vi "Data_Save_BOOST.vi"(9 "Data":T1) -> (2 "BOOST":string[](array[string]))   [LabVIEW 2017]
uses:
  Ctrls/Data.ctl
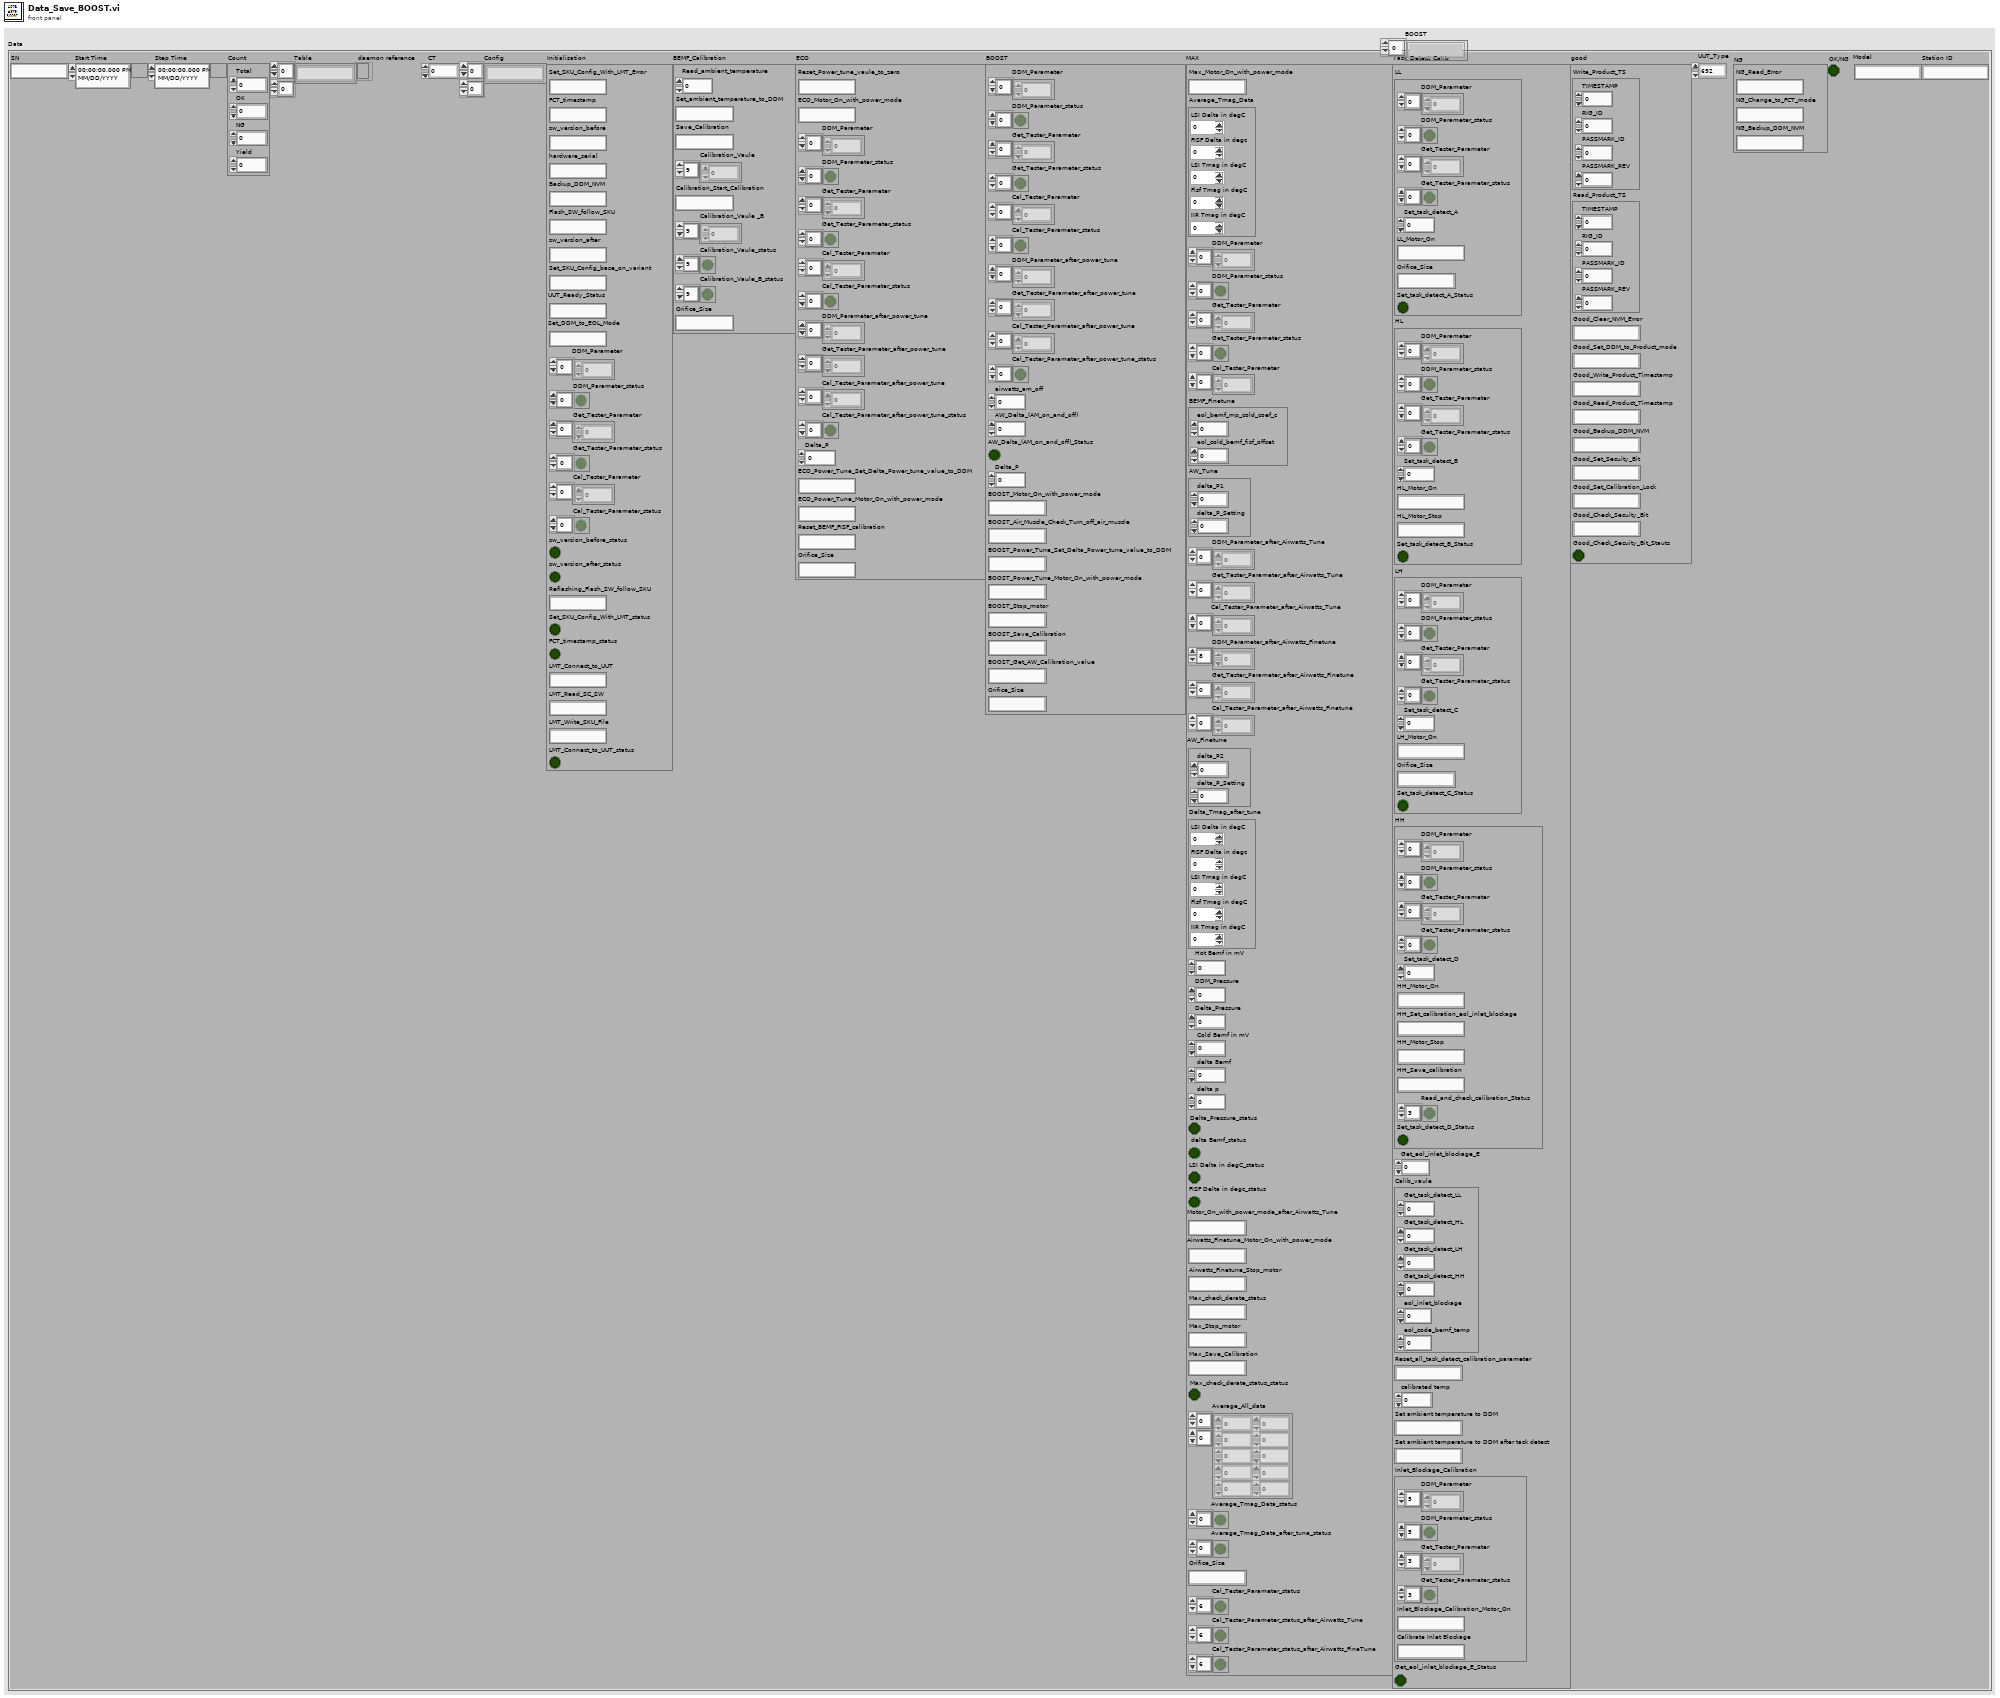
[diagram p1: front panel]
types:
  T1 = typedef "Data.ctl" = cluster{"SN":string, "Start Time":timestamp, "Step Time":timestamp, "Count":cluster{"Total":i32, "OK":i32, "NG":i32, "Yield":dbl}, "Table":string[][], "daemon reference":refnum<k5>, "CT":dbl, "Config":string[][], "Initialisation":cluster{"Set_SKU_Config_With_LMT_Error":string, "FCT_timestamp":string, "sw_version_before":string, "hardware_serial":string, "Backup_DDM_NVM":string, "Flash_SW_follow_SKU":string, "sw_version_after":string, "Set_SKU_Config_base_on_variant":string, "UUT_Ready_Status":string, "Set_DDM_to_EOL_Mode":string, "DDM_Parameter":dbl[], "DDM_Parameter_status":bool[], "Get_Tester_Parameter":dbl[], "Get_Tester_Parameter_status":bool[], "Cal_Tester_Parameter":dbl[], "Cal_Tester_Parameter_status":bool[], "sw_version_before_status":bool, "sw_version_after_status":bool, "Reflashing_Flash_SW_follow_SKU":string, "Set_SKU_Config_With_LMT_status":bool, "FCT_timestamp_status":bool, "LMT_Connect_to_UUT":string, "LMT_Read_SC_SW":string, "LMT_Write_SKU_File":string, "LMT_Connect_to_UUT_status":bool}, "BEMF_Calibration":cluster{"Read_ambient_temperature":dbl, "Set_ambient_temperature_to_DDM":string, "Save_Calibration":string, "Calibration_Vaule":dbl[], "Calibration_Start_Calibration":string, "Calibration_Vaule _B":dbl[], "Calibration_Vaule_status":bool[], "Calibration_Vaule_B_status":bool[], "Orifice_Size":string}, "ECO":cluster{"Reset_Power_tune_vaule_to_zero":string, "ECO_Motor_On_with_power_mode":string, "DDM_Parameter":dbl[], "DDM_Parameter_status":bool[], "Get_Tester_Parameter":dbl[], "Get_Tester_Parameter_status":bool[], "Cal_Tester_Parameter":dbl[], "Cal_Tester_Parameter_status":bool[], "DDM_Parameter_after_power_tune":dbl[], "Get_Tester_Parameter_after_power_tune":dbl[], "Cal_Tester_Parameter_after_power_tune":dbl[], "Cal_Tester_Parameter_after_power_tune_status":bool[], "Delta_P":dbl, "ECO_Power_Tune_Set_Delta_Power_tune_value_to_DDM":string, "ECO_Power_Tune_Motor_On_with_power_mode":string, "Reset_BEMF_FISF_calibration":string, "Orifice_Size":string}, "BOOST":cluster{"DDM_Parameter":dbl[], "DDM_Parameter_status":bool[], "Get_Tester_Parameter":dbl[], "Get_Tester_Parameter_status":bool[], "Cal_Tester_Parameter":dbl[], "Cal_Tester_Parameter_status":bool[], "DDM_Parameter_after_power_tune":dbl[], "Get_Tester_Parameter_after_power_tune":dbl[], "Cal_Tester_Parameter_after_power_tune":dbl[], "Cal_Tester_Parameter_after_power_tune_status":bool[], "airwatts_am_off":dbl, "AW_Delta_(AM_on_and_off)":dbl, "AW_Delta_(AM_on_and_off)_Status":bool, "Delta_P":dbl, "BOOST_Motor_On_with_power_mode":string, "BOOST_Air_Muscle_Check_Turn_off_air_muscle":string, "BOOST_Power_Tune_Set_Delta_Power_tune_value_to_DDM":string, "BOOST_Power_Tune_Motor_On_with_power_mode":string, "BOOST_Stop_motor":string, "BOOST_Save_Calibration":string, "BOOST_Get_AW_Calibration_value":string, "Orifice_Size":string}, "MAX":cluster{"Max_Motor_On_with_power_mode":string, "Average_Tmag_Data":cluster{"LSI Delta in degC":dbl, "FISF Delta in degc":dbl, "LSI Tmag in degC":dbl, "Fisf Tmag in degC":dbl, "IIR Tmag in degC":dbl}, "DDM_Parameter":dbl[], "DDM_Parameter_status":bool[], "Get_Tester_Parameter":dbl[], "Get_Tester_Parameter_status":bool[], "Cal_Tester_Parameter":dbl[], "BEMF_Finetune":cluster{"eol_bemf_mp_cold_coef_c":dbl, "eol_cold_bemf_fisf_offset":dbl}, "AW_Tune":cluster{"delta_P1":dbl, "delta_P_Setting":dbl}, "DDM_Parameter_after_Airwatts_Tune":dbl[], "Get_Tester_Parameter_after_Airwatts_Tune":dbl[], "Cal_Tester_Parameter_after_Airwatts_Tune":dbl[], "DDM_Parameter_after_Airwatts_Finetune":dbl[], "Get_Tester_Parameter_after_Airwatts_Finetune":dbl[], "Cal_Tester_Parameter_after_Airwatts_Finetune":dbl[], "AW_Finetune":cluster{"delta_P2":dbl, "delta_P_Setting":dbl}, "Delta_Tmag_after_tune":cluster{"LSI Delta in degC":dbl, "FISF Delta in degc":dbl, "LSI Tmag in degC":dbl, "Fisf Tmag in degC":dbl, "IIR Tmag in degC":dbl}, "Hot Bemf in mV":dbl, "DDM_Pressure":dbl, "Delta_Pressure":dbl, " Cold Bemf in mV":dbl, " delta Bemf":dbl, " delta p":dbl, "Delta_Pressure_status":bool, " delta Bemf_status":bool, "LSI Delta in degC_status":bool, "FISF Delta in degc_status":bool, "Motor_On_with_power_mode_after_Airwatts_Tune":string, "Airwatts_Finetune_Motor_On_with_power_mode":string, "Airwatts_Finetune_Stop_motor":string, "Max_check_derate_status":string, "Max_Stop_motor":string, "Max_Save_Calibration":string, "Max_check_derate_status_status":bool, "Average_All_data":dbl[][], "Average_Tmag_Data_status":bool[], "Average_Tmag_Data_after_tune_status":bool[], "Orifice_Size":string, "Cal_Tester_Parameter_status":bool[], "Cal_Tester_Parameter_status_after_Airwatts_Tune":bool[], "Cal_Tester_Parameter_status_after_Airwatts_FineTune":bool[]}, "Task_Detect_Calib":cluster{"LL":cluster{"DDM_Parameter":dbl[], "DDM_Parameter_status":bool[], "Get_Tester_Parameter":dbl[], "Get_Tester_Parameter_status":bool[], "Set_task_detect_A":dbl, "LL_Motor_On":string, "Orifice_Size":string, "Set_task_detect_A_Status":bool}, "HL":cluster{"DDM_Parameter":dbl[], "DDM_Parameter_status":bool[], "Get_Tester_Parameter":dbl[], "Get_Tester_Parameter_status":bool[], "Set_task_detect_B":dbl, "HL_Motor_On":string, "HL_Motor_Stop":string, "Set_task_detect_B_Status":bool}, "LH":cluster{"DDM_Parameter":dbl[], "DDM_Parameter_status":bool[], "Get_Tester_Parameter":dbl[], "Get_Tester_Parameter_status":bool[], "Set_task_detect_C":dbl, "LH_Motor_On":string, "Orifice_Size":string, "Set_task_detect_C_Status":bool}, "HH":cluster{"DDM_Parameter":dbl[], "DDM_Parameter_status":bool[], "Get_Tester_Parameter":dbl[], "Get_Tester_Parameter_status":bool[], "Set_task_detect_D":dbl, "HH_Motor_On":string, "HH_Set_calibration_eol_inlet_blockage":string, "HH_Motor_Stop":string, "HH_Save_calibration":string, "Read_and_check_calibration_Status":bool[], "Set_task_detect_D_Status":bool}, "Get_eol_inlet_blockage_E":dbl, "Calib_vaule":cluster{"Get_task_detect_LL":dbl, "Get_task_detect_HL":dbl, "Get_task_detect_LH":dbl, "Get_task_detect_HH":dbl, "eol_inlet_blockage":dbl, "eol_code_bemf_temp":dbl}, "Reset_all_task_detect_calibration_parameter":string, "calibrated temp":dbl, "Set ambient temperature to DDM":string, "Set ambient temperature to DDM after task detect":string, "Inlet_Blockage_Calibration":cluster{"DDM_Parameter":dbl[], "DDM_Parameter_status":bool[], "Get_Tester_Parameter":dbl[], "Get_Tester_Parameter_status":bool[], "Inlet_Blockage_Calibration_Motor_On":string, "Calibrate Inlet Blockage":string}, "Get_eol_inlet_blockage_E_Status":bool}, "good":cluster{"Write_Product_TS":cluster{"TIMESTAMP":i64, "RIG_ID":i64, "PASSMARK_ID":i64, "PASSMARK_REV":i64}, "Read_Product_TS":cluster{"TIMESTAMP":i64, "RIG_ID":i64, "PASSMARK_ID":i64, "PASSMARK_REV":i64}, "Good_Clear_NVM_Error":string, "Good_Set_DDM_to_Product_mode":string, "Good_Write_Product_Timestamp":string, "Good_Read_Product_Timestamp":string, "Good_Backup_DDM_NVM":string, "Good_Set_Secuity_Bit":string, "Good_Set_Calibration_Lock":string, "Good_Check_Secuity_Bit":string, "Good_Check_Secuity_Bit_Stauts":bool}, "UUT_Type":enum16{"692", "692B", "692D"}, "NG":cluster{"NG_Read_Error":string, "NG_Change_to_FCT_mode":string, "NG_Backup_DDM_NVM":string}, "OK/NG":bool, "Model":string, "Station ID":string}
  T2 = typedef "HD Config.ctl" = cluster{" PC":cluster{"PC Address":u8[], "PC Port":i32}, "FCO":cluster{"COM":refnum<visa-resource-name>, "Baudrate":u32}, "DC Power ":cluster{"COM":refnum<visa-resource-name>, "Baudrate":u32}, "PW3336":cluster{"COM":refnum<visa-resource-name>, "Baudrate":u32}, "Lefoo":cluster{"COM":refnum<visa-resource-name>, "Baudrate":u32}, "AI Model":cluster{"COM":refnum<visa-resource-name>, "Baudrate":u32}, "DIPC":cluster{"COM":refnum<visa-resource-name>}, "Daemon":cluster{"IP Address":string, "Port":u16, "Retry":u16}, "Motor":cluster{"COM":refnum<visa-resource-name>, "Baudrate":u32}, "G1":bool, "Fail_resume_mode":bool, "Skip DDM Speed&Pressure Passmark":bool}
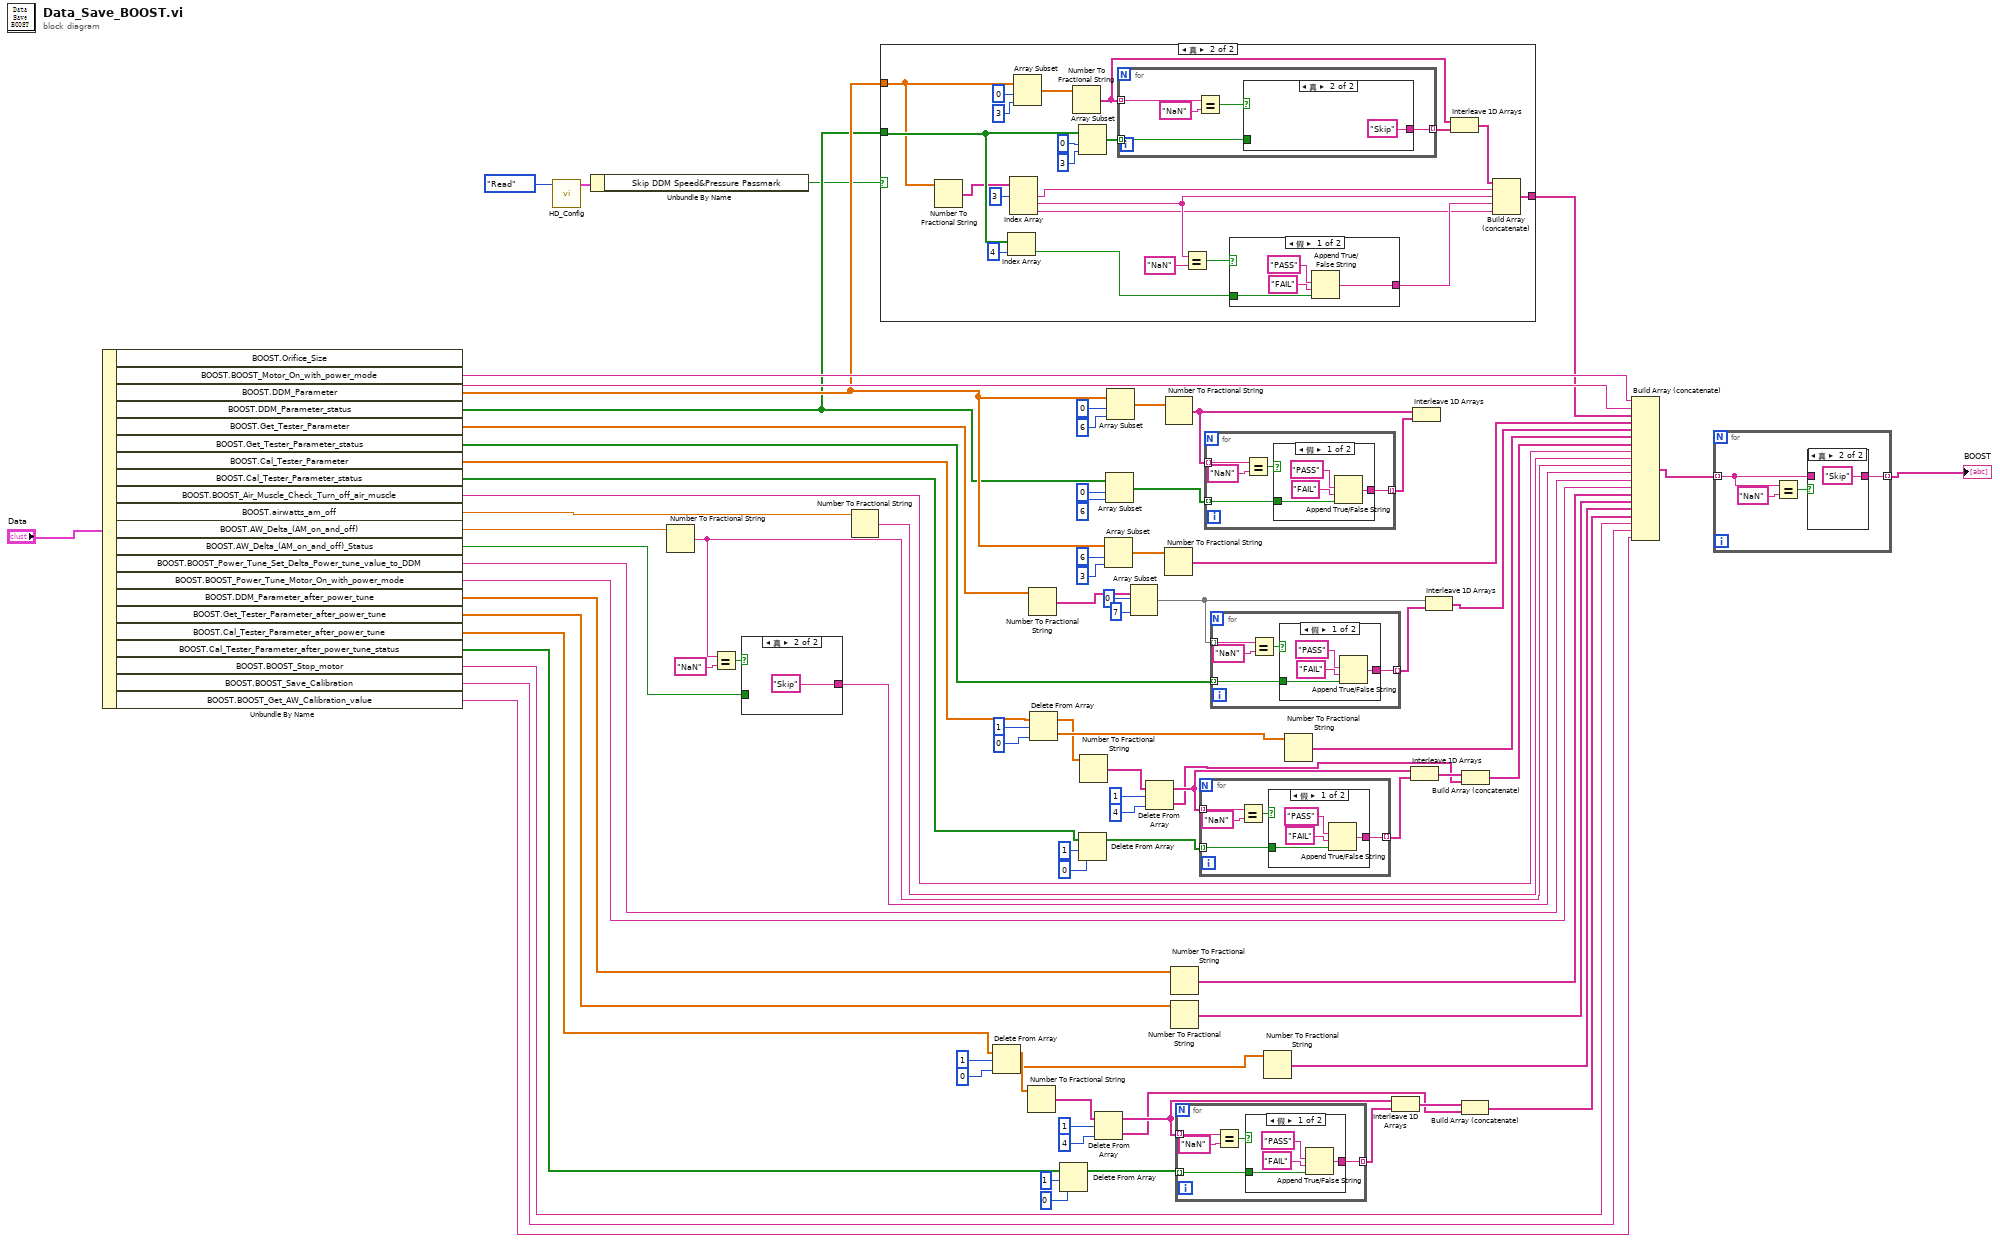
[diagram p0: block diagram]
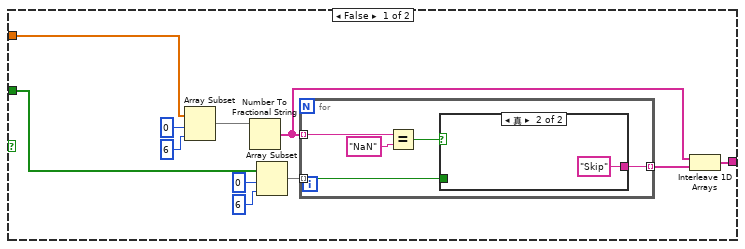
[diagram p2: hidden frame]
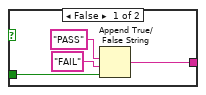
[diagram p3: hidden frame]
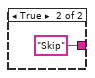
[diagram p4: hidden frame]
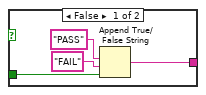
[diagram p5: hidden frame]
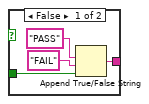
[diagram p6: hidden frame]
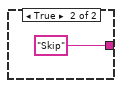
[diagram p8: hidden frame]
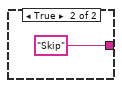
[diagram p9: hidden frame]
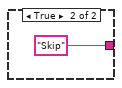
[diagram p10: hidden frame]
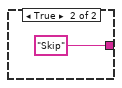
[diagram p11: hidden frame]
diagram:
  n1 = Unbundle By Name("Data") -> ("BOOST.Orifice_Size"=w25:string, "BOOST.BOOST_Motor_On_with_power_mode"=w26:string, "BOOST.DDM_Parameter"=w24:dbl[], "BOOST.DDM_Parameter_status"=w23:bool[], "BOOST.Get_Tester_Parameter"=w14:dbl[], "BOOST.Get_Tester_Parameter_status"=w38:bool[], "BOOST.Cal_Tester_Parameter"=w65:dbl[], "BOOST.Cal_Tester_Parameter_status"=w64:bool[], "BOOST.BOOST_Air_Muscle_Check_Turn_off_air_muscle"=w51:string, "BOOST.airwatts_am_off"=w50:dbl, "BOOST.AW_Delta_(AM_on_and_off)"=w49:dbl, "BOOST.AW_Delta_(AM_on_and_off)_Status"=w29:bool, "BOOST.BOOST_Power_Tune_Set_Delta_Power_tune_value_to_DDM"=w47:string, "BOOST.BOOST_Power_Tune_Motor_On_with_power_mode"=w46:string, "BOOST.DDM_Parameter_after_power_tune"=w81:dbl[], "BOOST.Get_Tester_Parameter_after_power_tune"=w82:dbl[], "BOOST.Cal_Tester_Parameter_after_power_tune"=w55:dbl[], "BOOST.Cal_Tester_Parameter_after_power_tune_status"=w54:bool[], "BOOST.BOOST_Stop_motor"=w45:string, "BOOST.BOOST_Save_Calibration"=w44:string, "BOOST.BOOST_Get_AW_Calibration_value"=w43:string)
  n2 = call "HD_Config.vi"("Step"=enum16{"Initial", "Write", "Read"}."Read") -> ("HD Config out"=w20:T2)  [unwired: 9 in, 1 out]
  n3 = Unbundle By Name(w20) -> ("Skip DDM Speed&Pressure Passmark"=w19:bool)
  n4 = Number To Fractional String(number=w49) -> (F-format string=w28:string)  [unwired: 3 in]
  n5 = Equal?(x=w28, y="NaN" ("x")) -> (x = y?=w30:bool)
  n6 = case shown="真" w30 {
    tunnel: w29 -> [w89 _]
    tunnel: [w87 "Skip" ("x")] -> w27
    frame False {
      n7 = Append True/False String(1:w89, 2:"FAIL" ("字符串(\"\")"), 3:"PASS" ("真字符串")) -> (0:w87:string)  [unwired: 1 in]
    }
    frame True {
    }
  }
  n8 = Number To Fractional String(number=w50) -> (F-format string=w48:string)  [unwired: 3 in]
  n9 = case shown="真" w19 {
    tunnel: w23 -> [w92 w123]
    tunnel: w24 -> [w93 w120]
    tunnel: [w91 w112] -> w22
    frame False {
      n10 = Array Subset(array=w93, index=0 ("索引"), length=6 ("长度")) -> (w99:dbl[])
      n11 = Number To Fractional String(number=w99) -> (F-format string=w98:string[])  [unwired: 3 in]
      n12 = Array Subset(array=w92, index=0 ("索引"), length=6 ("长度")) -> (w100:bool[])
      n13 = for {
        tunnel: w100 -> [w106] mode=indexing
        tunnel: [w105] -> w101 mode=indexing
        tunnel: w98 -> [w103] mode=indexing
        n14 = Equal?(x=w103, y="NaN" ("x")) -> (x = y?=w102:bool)
        n15 = case shown="真" w102 {
          tunnel: w106 -> [w110 _]
          tunnel: [w108 "Skip" ("x")] -> w105
          frame False {
            n16 = Append True/False String(1:w110, 2:"FAIL" ("字符串(\"\")"), 3:"PASS" ("真字符串")) -> (0:w108:string)  [unwired: 1 in]
          }
          frame True {
          }
        }
      }
      n17 = Interleave 1D Arrays(w98, w101) -> (w91:string[])
    }
    frame True {
      n18 = Number To Fractional String(number=w120) -> (F-format string=w119:string[])  [unwired: 3 in]
      n19 = Index Array(array=w123, index=4 ("索引")) -> (element=w118:bool)
      n20 = Index Array(array=w119, index #1=3 ("索引")) -> (element #1=w117:string, element #2=w115:string, element #3=w114:string)  [unwired: 2 in]
      n21 = Array Subset(array=w120, index=0 ("索引"), length=3 ("长度")) -> (w131:dbl[])
      n22 = Number To Fractional String(number=w131) -> (F-format string=w126:string[])  [unwired: 3 in]
      n23 = Array Subset(array=w123, index=0 ("索引"), length=3 ("长度")) -> (w132:bool[])
      n24 = for {
        tunnel: w132 -> [w143] mode=indexing
        tunnel: [w142] -> w133 mode=indexing
        tunnel: w126 -> [w140] mode=indexing
        n25 = Equal?(x=w140, y="NaN" ("x")) -> (x = y?=w139:bool)
        n26 = case shown="真" w139 {
          tunnel: w143 -> [w147 _]
          tunnel: [w145 "Skip" ("x")] -> w142
          frame False {
            n27 = Append True/False String(1:w147, 2:"FAIL" ("字符串(\"\")"), 3:"PASS" ("真字符串")) -> (0:w145:string)  [unwired: 1 in]
          }
          frame True {
          }
        }
      }
      n28 = Equal?(x=w115, y="NaN" ("x")) -> (x = y?=w122:bool)
      n29 = case shown="假" w122 {
        tunnel: w118 -> [w137 _]
        tunnel: [w135 "Skip" ("x")] -> w116
        frame False {
          n30 = Append True/False String(1:w137, 2:"FAIL" ("字符串(\"\")"), 3:"PASS" ("真字符串")) -> (0:w135:string)  [unwired: 1 in]
        }
        frame True {
        }
      }
      n31 = Interleave 1D Arrays(w126, w133) -> (w113:string[])
      n32 = Build Array (concatenate)(w113, w117, w115, w116, w114) -> (w112:string[])
    }
  }
  n33 = Delete From Array(array=w55, length=1 ("长度"), index=0 ("索引")) -> (deleted portion=w58:dbl[], array with subset deleted=w59:dbl[])
  n34 = Number To Fractional String(number=w59) -> (F-format string=w4:string[])  [unwired: 3 in]
  n35 = Number To Fractional String(number=w14) -> (F-format string=w15:string[])  [unwired: 3 in]
  n36 = Delete From Array(array=w65, length=1 ("长度"), index=0 ("索引")) -> (deleted portion=w69:dbl[], array with subset deleted=w68:dbl[])
  n37 = Delete From Array(array=w54, length=1 ("长度"), index=0 ("索引")) -> (array with subset deleted=w35:bool[])  [unwired: 1 out]
  n38 = Delete From Array(array=w64, length=1 ("长度"), index=0 ("索引")) -> (array with subset deleted=w36:bool[])  [unwired: 1 out]
  n39 = Number To Fractional String(number=w68) -> (F-format string=w11:string[])  [unwired: 3 in]
  n40 = Delete From Array(array=w4, length=1 ("长度"), index=4 ("索引")) -> (deleted portion=w1:string[], array with subset deleted=w3:string[])
  n41 = Array Subset(array=w24, index=6 ("索引"), length=3 ("长度")) -> (w73:dbl[])
  n42 = Array Subset(array=w23, index=0 ("索引"), length=6 ("长度")) -> (w41:bool[])
  n43 = Array Subset(array=w24, index=0 ("索引"), length=6 ("长度")) -> (w74:dbl[])
  n44 = Array Subset(array=w15, index=0 ("索引"), length=7 ("长度")) -> (w18:string[])
  n45 = Delete From Array(array=w11, length=1 ("长度"), index=4 ("索引")) -> (deleted portion=w8:string[], array with subset deleted=w10:string[])
  n46 = Number To Fractional String(number=w73) -> (F-format string=w83:string[])  [unwired: 3 in]
  n47 = Number To Fractional String(number=w74) -> (F-format string=w40:string[])  [unwired: 3 in]
  n48 = Number To Fractional String(number=w81) -> (F-format string=w84:string[])  [unwired: 3 in]
  n49 = Number To Fractional String(number=w82) -> (F-format string=w85:string[])  [unwired: 3 in]
  n50 = for {
    tunnel: w35 -> [w153] mode=indexing
    tunnel: [w152] -> w34 mode=indexing
    tunnel: w3 -> [w150] mode=indexing
    n51 = Equal?(x=w150, y="NaN" ("x")) -> (x = y?=w149:bool)
    n52 = case shown="假" w149 {
      tunnel: w153 -> [w157 _]
      tunnel: [w155 "Skip" ("x")] -> w152
      frame False {
        n53 = Append True/False String(1:w157, 2:"FAIL" ("字符串(\"\")"), 3:"PASS" ("真字符串")) -> (0:w155:string)  [unwired: 1 in]
      }
      frame True {
      }
    }
  }
  n54 = for {
    tunnel: w36 -> [w163] mode=indexing
    tunnel: [w162] -> w37 mode=indexing
    tunnel: w10 -> [w160] mode=indexing
    n55 = Equal?(x=w160, y="NaN" ("x")) -> (x = y?=w159:bool)
    n56 = case shown="假" w159 {
      tunnel: w163 -> [w167 _]
      tunnel: [w165 "Skip" ("x")] -> w162
      frame False {
        n57 = Append True/False String(1:w167, 2:"FAIL" ("字符串(\"\")"), 3:"PASS" ("真字符串")) -> (0:w165:string)  [unwired: 1 in]
      }
      frame True {
      }
    }
  }
  n58 = for {
    tunnel: w41 -> [w173] mode=indexing
    tunnel: [w172] -> w42 mode=indexing
    tunnel: w40 -> [w170] mode=indexing
    n59 = Equal?(x=w170, y="NaN" ("x")) -> (x = y?=w169:bool)
    n60 = case shown="假" w169 {
      tunnel: w173 -> [w177 _]
      tunnel: [w175 "Skip" ("x")] -> w172
      frame False {
        n61 = Append True/False String(1:w177, 2:"FAIL" ("字符串(\"\")"), 3:"PASS" ("真字符串")) -> (0:w175:string)  [unwired: 1 in]
      }
      frame True {
      }
    }
  }
  n62 = for {
    tunnel: w38 -> [w183] mode=indexing
    tunnel: [w182] -> w39 mode=indexing
    tunnel: w18 -> [w180] mode=indexing
    n63 = Equal?(x=w180, y="NaN" ("x")) -> (x = y?=w179:bool)
    n64 = case shown="假" w179 {
      tunnel: w183 -> [w187 _]
      tunnel: [w185 "Skip" ("x")] -> w182
      frame False {
        n65 = Append True/False String(1:w187, 2:"FAIL" ("字符串(\"\")"), 3:"PASS" ("真字符串")) -> (0:w185:string)  [unwired: 1 in]
      }
      frame True {
      }
    }
  }
  n66 = Number To Fractional String(number=w58) -> (F-format string=w53:string[])  [unwired: 3 in]
  n67 = Number To Fractional String(number=w69) -> (F-format string=w63:string[])  [unwired: 3 in]
  n68 = Interleave 1D Arrays(w3, w34) -> (w52:string[])
  n69 = Interleave 1D Arrays(w10, w37) -> (w62:string[])
  n70 = Interleave 1D Arrays(w40, w42) -> ()  [unwired: 1 out]
  n71 = Interleave 1D Arrays(w18, w39) -> (w7:string[])
  n72 = Build Array (concatenate)(w52, w1) -> (w2:string[])
  n73 = Build Array (concatenate)(w62, w8) -> (w9:string[])
  n74 = Build Array (concatenate)(w25, w26, w22, w83, w7, w63, w9, w51, w48, w28, w27, w47, w46, w84, w85, w53, w2, w45, w44, w43) -> (w33:string[])
  n75 = for {
    tunnel: [w192] -> w32 mode=indexing
    tunnel: w33 -> [w189] mode=indexing
    n76 = Equal?(x=w189, y="NaN" ("x")) -> (x = y?=w190:bool)
    n77 = case shown="真" w190 {
      tunnel: [w193 "Skip" ("x")] -> w192
      tunnel: w189 -> [w193 _]
      frame False {
      }
      frame True {
      }
    }
  }
  "BOOST" <- w32
